vi "UserVars-Fill Table.vi"(10 "UserVars":T1[](array[typedef]), 11 ".NET Refnum":refnum<k24>) -> ()   [LabVIEW 2015]
uses:
  D:/Experiment VIs/Utility VIs/User Variables/dotNET Source/UserVariableControls/bin/Release/UserVariableControls.dll
  dotNET Source/UserVariableControls/bin/Release/UserVariableControls.dll
  User Variable.ctl
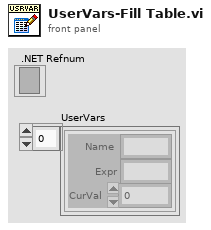
[diagram p1: front panel]
types:
  T1 = typedef "User Variable.ctl" = cluster{"Name":string, "Expr":string, "CurVal":dbl}
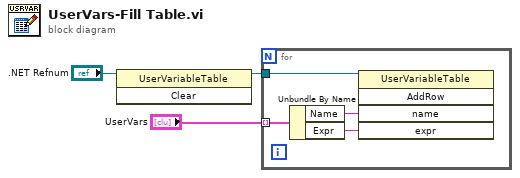
[diagram p0: block diagram]
diagram:
  n1 = invoke class="UserVariableTable" method="Clear"(reference=".NET Refnum") -> (reference out=w2:refnum<k24>)  [unwired: 2 in, 2 out]
  n2 = for {
    tunnel: w2 -> [w7]
    tunnel: "UserVars" -> [w6] mode=indexing
    n3 = Unbundle By Name(w6) -> ("Name"=w5:string, "Expr"=w4:string)
    n4 = invoke class="UserVariableTable" method="AddRow"(reference=w7, "name"=w5, "expr"=w4) -> ()  [unwired: 2 in, 5 out]
  }
